vi "RefereeVSS.vi"(6 "RX":bool, 11 "element":u8[](array[numeric])) -> (0 "error out 2":errorcluster, 3 "output cluster":T2)   [LabVIEW 2020]
uses:
  vss/SSL_AI/Vision_class/Old vision/Controls/SSL Referee.ctl
  vss/SSL_AI/Vision_class/Old vision/Decode SSL and Refree Wrapper Package Folder/SSL Referee Team Info.ctl
  vss/SSL_AI/Vision_class/Old vision/Decode SSL and Refree Wrapper Package Folder/Varint Decoder uint32.vi
panel:
  out "Cluster":T1
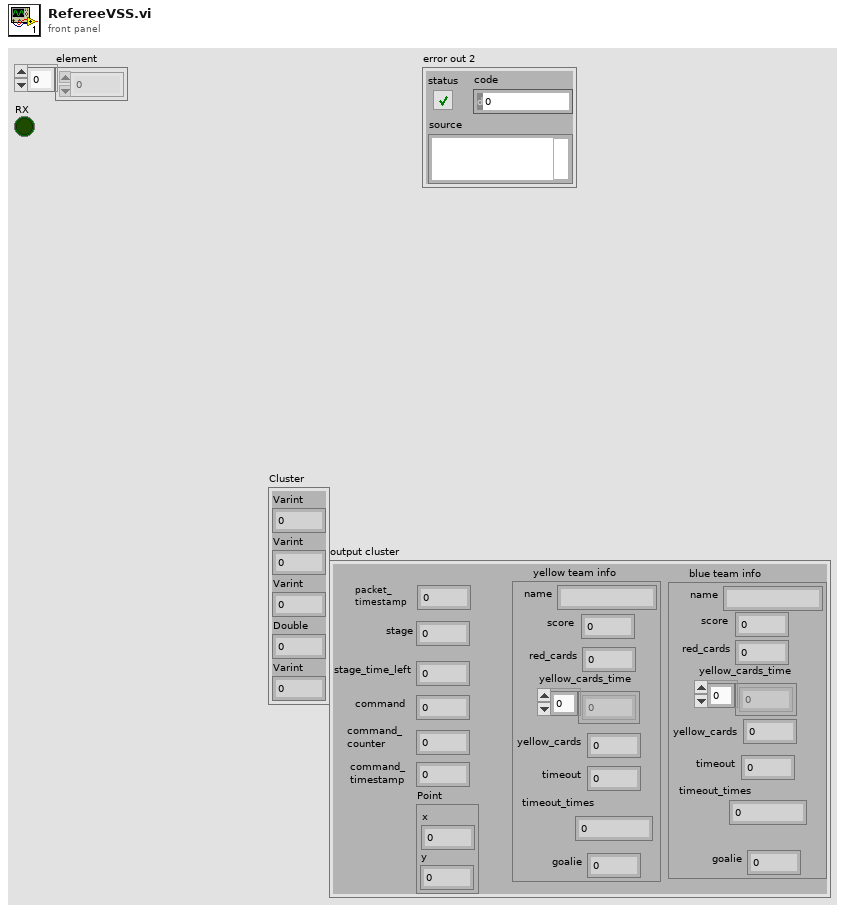
[diagram p1: front panel]
types:
  T1 = cluster{"Varint":u32, "Varint":u32, "Varint":u32, "Double":dbl, "Varint":u32}
  T2 = typedef "SSL Referee.ctl" = cluster{"packet_\ntimestamp":u64, "stage":u64, "stage_time_left":i32, "command ":u64, "command_\ncounter ":u32, "command_\ntimestamp":u64, "yellow team info":T3, "blue team info":T3, "Point":cluster{"x":sgl, "y":sgl}}
  T3 = typedef "SSL Referee Team Info.ctl" = cluster{"name":string, "score":u32, "red_cards":u32, "yellow_cards_time":u32[], "yellow_cards":u32, "timeout":u32, "timeout_times":u32, "goalie":u32}
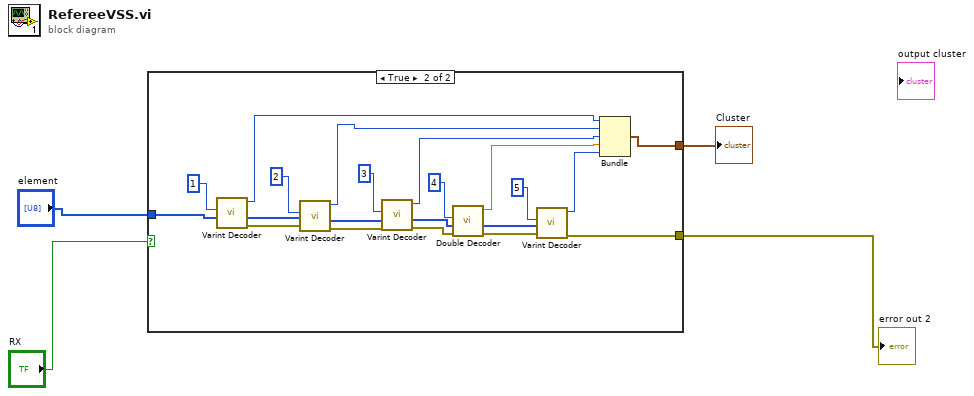
[diagram p0: block diagram]
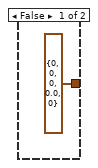
[diagram p2: hidden frame]
diagram:
  n1 = case shown="True" "RX" {
    tunnel: "element" -> [_ w26]
    tunnel: [T1 {"Varint"=0, "Varint"=0, "Varint"=0, "Double"=0.0, "Varint"=0} w7] -> w2
    tunnel: [_ w6] -> w1
    frame False {
    }
    frame True {
      n2 = call-poly "Varint Decoder.vi"("Array"=w26, "Key"=1) -> ("error out"=w16:errorcluster, "array w/ subset deleted"=w24:u8[], "Varint"=w12:u32)  [unwired: 6 in, 1 out]
      n3 = call-poly "Varint Decoder.vi"("error in (no error)"=w16, "Array"=w24, "Key"=2) -> ("error out"=w15:errorcluster, "array w/ subset deleted"=w22:u8[], "Varint"=w11:u32)  [unwired: 5 in, 1 out]
      n4 = call-poly "Varint Decoder.vi"("error in (no error)"=w15, "Array"=w22, "Key"=3) -> ("error out"=w14:errorcluster, "array w/ subset deleted"=w20:u8[], "Varint"=w10:u32)  [unwired: 5 in, 1 out]
      n5 = call "Double Decoder.vi"("error in (no error)"=w14, "Array"=w20, "Key"=4) -> ("error out"=w13:errorcluster, "array w/ subset deleted"=w18:u8[], "Double"=w9:dbl)  [unwired: 5 in, 1 out]
      n6 = call-poly "Varint Decoder.vi"("error in (no error)"=w13, "Array"=w18, "Key"=5) -> ("error out"=w6:errorcluster, "Varint"=w8:u32)  [unwired: 5 in, 2 out]
      n7 = Bundle("Varint"=w12, "Varint"=w11, "Varint"=w10, "Double"=w9, "Varint"=w8) -> (w7:T1)  [unwired: 1 in]
    }
  }
  "error out 2" <- w1
  "Cluster" <- w2
